vi "Set Group State Filter.vi"(10 "Group:State":string[](array[string]), 11 "GlobalLogFilter in":refnum<class "GlobalLogFilter.lvclass">) -> (3 "GlobalLogFilter out":refnum<class "GlobalLogFilter.lvclass">)   [LabVIEW 2017, in "GlobalLogFilter.lvclass"]
uses:
  GlobalLogFilter.lvclass
  GlobalLogFilter.lvclass/GlobalLogFilter.ctl
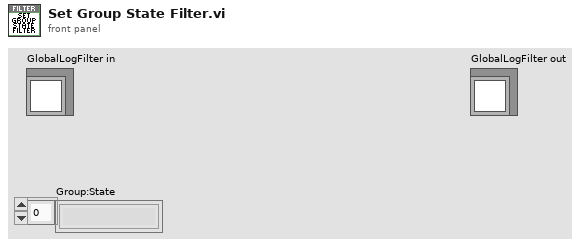
[diagram p1: front panel]
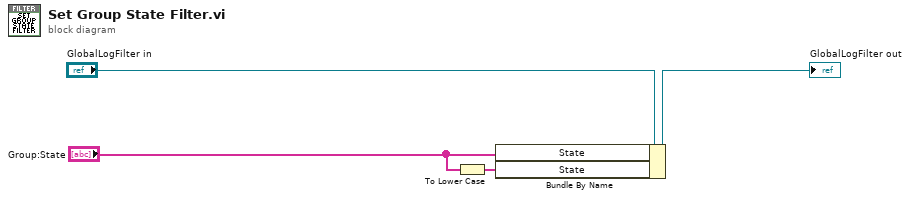
[diagram p0: block diagram]
diagram:
  n1 = To Lower Case(string="Group:State") -> (all lower case string=w1:string[])
  n2 = Bundle By Name(cluster="GlobalLogFilter in", "State"="Group:State", "State"=w1) -> (→"GlobalLogFilter out":refnum<class "GlobalLogFilter.lvclass">)
